vi "XBrio write test4 (flatten to string).vi"() -> ()   [LabVIEW 2013]
uses:
  C:/Program Files (x86)/National Instruments/LabVIEW 2013/examples/Instrument IO/Serial/support/Serial - Settings.ctl
  <vilib>/Instr/_visa.llb/VISA Configure Serial Port (Instr).vi
panel:
  out "appended array":u8[](array[numeric])
  in  "Number being sent 2":u8
  out "String being written in HEX":string
  out "String being written":string
  in  "Number being sent":u8
  out "Bytes being written":u32
  in  "VISA resource name":refnum<visa-resource-name>="COM1"
  in  "delay before read (ms)":u32=500
  out "bytes read":u32
  in  "Serial Settings":T1={"baud rate"=9600, "data bits"=8, "parity"=enum."None", "stop bits"=10, "flow control"=0} {"flow control" items=["None"=0, "XON/XOFF"=1, "RTS/CTS"=2, "DTR/DSR"=4]; "stop bits" items=["1.0"=10, "1.5"=15, "2.0"=20]; "data bits" min=5 max=8 step=1; "baud rate" items=["75"=75, "110"=110, "134"=134, "150"=150, "300"=300, "600"=600, "1200"=1200, "1800"=1800, "2400"=2400, "4800"=4800, "7200"=7200, "9600"=9600, "14400"=14400, "19200"=19200, "28800"=28800, "38400"=38400, "56000"=56000, "57600"=57600, "115200"=115200, "128000"=128000, "230400"=230400]}
  in  "?":bool
  out "Response":string
  out "String to U16":u16[](array[numeric])
  out "IR2":u16
  out "IR1":u16
  out "Encoder1":u16
  out "Encoder2":u16
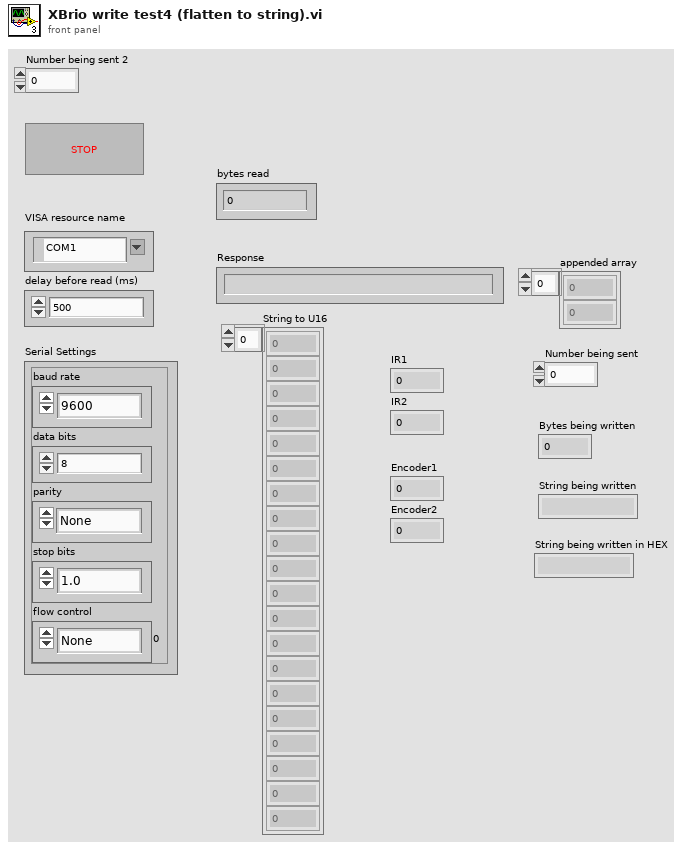
[diagram p1: front panel]
types:
  T1 = typedef "Serial - Settings.ctl" = cluster{"baud rate":u32, "data bits":u16, "parity":enum16{"None", "Odd", "Even", "Mark", "Space"}, "stop bits":u16, "flow control":u16}
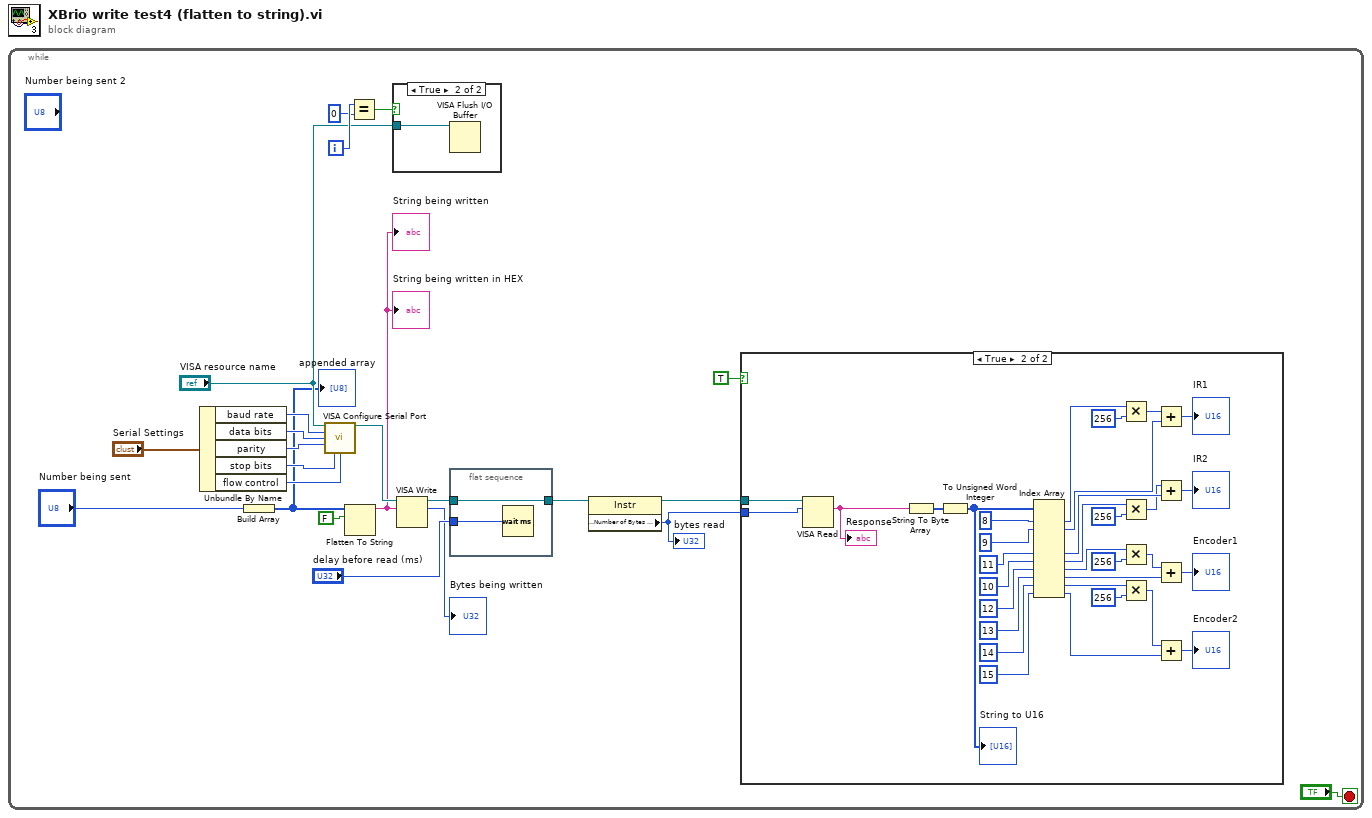
[diagram p0: block diagram]
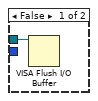
[diagram p2: hidden frame]
diagram:
  n1 = while {
    i -> [w14]
    stop <- "?" stop-if-true
    n2 = Unbundle By Name("Serial Settings") -> ("baud rate"=w21:u32, "data bits"=w20:u16, "parity"=w19:enum16{"None", "Odd", "Even", "Mark", "Space"}, "stop bits"=w18:u16, "flow control"=w17:u16)
    n3 = Build Array("Number being sent") -> (w2:u8[])
    "appended array" <- w2
    n4 = call-poly "VISA Configure Serial Port"("VISA resource name"="VISA resource name", "baud rate (9600)"=w21, "data bits (8)"=w20, "parity (0:none)"=w19, "stop bits (10: 1 bit)"=w18, "flow control (0:none)"=w17) -> ("VISA resource name out"=w8:refnum<visa-resource-name>)  [unwired: 3 in, 6 out]
    n5 = Flatten To String(anything=w2, prepend array or string size? (T)=FALSE) -> (data string=w3:string)  [unwired: 2 in, 2 out]
    "String being written" <- w3
    "String being written in HEX" <- w3
    n6 = Equal?(x=w14, y=0) -> (x = y?=w12:bool)
    n7 = case shown="True" w12 {
      tunnel: "VISA resource name" -> [_ w58]
      frame False {
      }
      frame True {
        n8 = VISA Flush I/O Buffer(VISA resource name=w58) -> ()  [unwired: 2 in, 2 out]
      }
    }
    n9 = VISA Write(VISA resource name=w8, write buffer=w3) -> (VISA resource name out=w7:refnum<visa-resource-name>, return count=→"Bytes being written":u32)  [unwired: 1 in, 1 out]
    n10 = flat-sequence {
      tunnel: w7 -> [w59]
      tunnel: [w59] -> w16
      tunnel: "delay before read (ms)" -> [w60]
      frame #0 {
        n11 = Wait (ms)(milliseconds to wait=w60) -> ()  [unwired: 1 out]
      }
    }
    n12 = property class="Instr"(reference=w16) -> (reference out=w9:refnum<visa-resource-name>, "Serial Settings:Number of Bytes at Serial Port"=w10:u32)  [unwired: 1 in, 1 out]
    "bytes read" <- w10
    n13 = case shown="True" TRUE {
      tunnel: w10 -> [_ w26]
      tunnel: w9 -> [w24 w25]
      frame False {
        n14 = VISA Flush I/O Buffer(VISA resource name=w24) -> ()  [unwired: 2 in, 2 out]
      }
      frame True {
        n15 = VISA Read(VISA resource name=w25, byte count=w26) -> (read buffer=w28:string)  [unwired: 1 in, 3 out]
        "Response" <- w28
        n16 = String To Byte Array(string=w28) -> (unsigned byte array=w29:u8[])
        n17 = To Unsigned Word Integer(number=w29) -> (unsigned 16bit integer=w27:u16[])
        "String to U16" <- w27
        n18 = Index Array(array=w27, index #1=8 ("index"), index #2=9 ("index"), index #5=11, index #6=10 ("index"), index #7=12 ("index"), index #8=13 ("index"), index #9=14 ("index"), index #10=15 ("index")) -> (element #1=w37:u16, element #2=w40:u16, element #5=w34:u16, element #6=w32:u16, element #7=w45:u16, element #8=w46:u16, element #9=w52:u16, element #10=w53:u16)  [unwired: 2 in, 2 out]
        n19 = Multiply(x=w37, y=u16 256) -> (x*y=w39:u16)
        n20 = Multiply(x=w32, y=u16 256) -> (x*y=w30:u16)
        n21 = Multiply(x=w45, y=u16 256) -> (x*y=w41:u16)
        n22 = Multiply(x=w52, y=u16 256) -> (x*y=w51:u16)
        n23 = Add(x=w39, y=w40) -> (x+y=→"IR1":u16)
        n24 = Add(x=w30, y=w34) -> (x+y=→"IR2":u16)
        n25 = Add(x=w41, y=w46) -> (x+y=→"Encoder1":u16)
        n26 = Add(x=w51, y=w53) -> (x+y=→"Encoder2":u16)
      }
    }
  }
